vi "Athena Command Main v3.vi"() -> ()   [LabVIEW 2009]
uses:
  UDP3-GPS, INS/UDP 3.ctl
  UDP3-GPS, INS/UDP3rtglob.vi
  <vilib>/userDefined/High Color/nirio_resource_hc.ctl
  <vilib>/rvi/interface/nirviOpenFPGA/nirviOpenFPGA.xnode
  FPGA Bitfiles/Athena Brain.lvproj_FPGA Target 2_FPGA Main.vi.lvbitx
  <vilib>/FPGAPlugInAG/sbRIO-9642/nirviIntfOpen_sbRIO-9642.vi
  <vilib>/rvi/interface/nirviReadWriteControl/nirviReadWriteControl.xnode
  <vilib>/Utility/error.llb/Error Cluster From Error Code.vi
  <vilib>/rvi/errors/niLvFpgaAdjustHostInterfaceError.vi
  <vilib>/rvi/interface/common/niFpgaNodeNameForErrorReporting.ctl
  <vilib>/rvi/errors/niLvFpgaWhatHappensToTopLevelVI.ctl
  <vilib>/LabVIEW Targets/FPGA/RIO/nirio_HostInterface/nirio_ReadBig.vi
  <vilib>/rvi/interface/nirviCloseFPGA/nirviCloseFPGA.xnode
  <vilib>/FPGAPlugInAG/sbRIO-9642/nirviIntfClose_sbRIO-9642.vi
  NiRioSrv.dll
panel:
  out "UDP 3":T1
  in  "Waypoints":cluster{"Latitude":dbl, "Longitude":dbl}[](array[cluster])=[{"Latitude"=42.294143531505355, "Longitude"=-71.26439183950424}, {"Latitude"=42.294083018570596, "Longitude"=-71.2644910812378}, {"Latitude"=42.2940443299425, "Longitude"=-71.2644575536251}, {"Latitude"=42.29408698663367, "Longitude"=-71.26439049839973}]
  out "Heartbeat":bool
  in  "Waypoint Heading":i8
  in  "stop":bool
  in  "Autonomus?":bool=TRUE
  in  "Steering Position Offset":i32
  in  "Steering Control Gain":fxp<+/-,20,5>=0.149993896484375 format="%.17g"
  out "Steering Enabled":bool
  out "Drive Enabled":bool
  out "Speed":dbl(knob) scale=0.0..10.0
  out "Meter":i32(knob) scale=-35.0..35.0
  in  "Tab Control":enum32{"Human Control", "Autonomous"}(tab)=enum."Autonomous"
  in  "Drive Enable":bool
  in  "Steering Enable":bool
  in  "Drive Speed Current (1-3.5)":fxp<+/-,18,8> format="%.13g"
  in  "Steering Position Target":i32
  out "Drive Encoder ft/sec":fxp<+/-,18,8> format="%.13g"
  out "Drivable Paths":T2(graph)
  out "obstacle driveable path lengths":u16[](array[numeric])
  out "line driveable path lengths":u16[](array[numeric])
  in  "min obstacle dist":u16
  in  "paths to graph":enum16{"lines", "obstacles", "both"}(ring)
  in  "Auton Drive Speed Current":fxp<+/-,18,8> format="%.13g"
  in  "obstacle proximity":i16=400
  in  "line proximity":i16=100
  out "Current Heading":cluster{"Lat":dbl, "Longe":dbl, "heading":dbl}
  in  "Override Objective Direction":i8=35
  in  "Use Both Vision and Obstacles":bool
  in  "Display Graph":bool=TRUE
  # "Autonomous"
  # "Human Control"
  # "-35"
  # "-30"
  # "-25"
  # "-20"
  # "-15"
  # "-10"
  # "-5"
  # "-1"
  # "1"
  # "5"
  # "10"
  # "15"
  # "20"
  # "25"
  # "30"
  # "35"
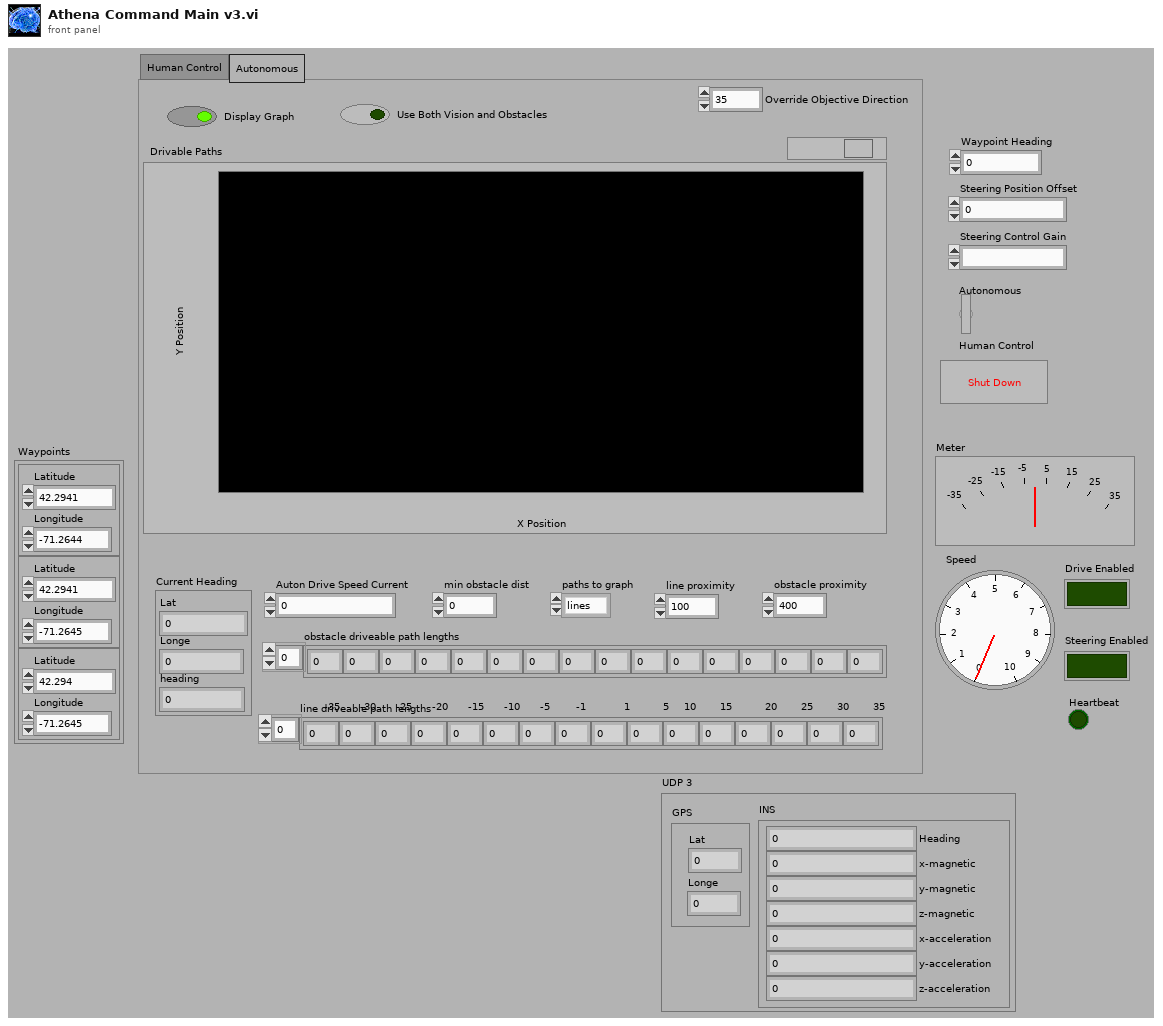
[diagram p1: front panel]
types:
  T1 = typedef "UDP 3.ctl" = cluster{"GPS":cluster{"Lat":dbl, "Longe":dbl}, "INS":cluster{"Heading":dbl, "x-magnetic":dbl, "y-magnetic":dbl, "z-magnetic":dbl, "x-acceleration":dbl, "y-acceleration":dbl, "z-acceleration":dbl}}
  T2 = cluster{"New X Position":i16, "New Y Position":i16}[]
  T3 = typedef "nirio_resource_hc.ctl" = tag
  T4 = typedef "niFpgaNodeNameForErrorReporting.ctl" = enum16{"Open FPGA VI Reference", "Read/Write Control", "Invoke Method: Abort", "Invoke Method: Acknowledge IRQ", "Invoke Method: Download", "Invoke Method: FIFO.Configure", "Invoke Method: FIFO.Read", "Invoke Method: FIFO.Start", "Invoke Method: FIFO.Stop", "Invoke Method: FIFO.Write", "Invoke Method: Reset", "Invoke Method: Run", "Invoke Method: Wait on IRQ", "Close FPGA VI Reference"}
  T5 = typedef "niLvFpgaWhatHappensToTopLevelVI.ctl" = enum16{"top level VI scripted behind XNode", "top level VI inlined behind XNode"}
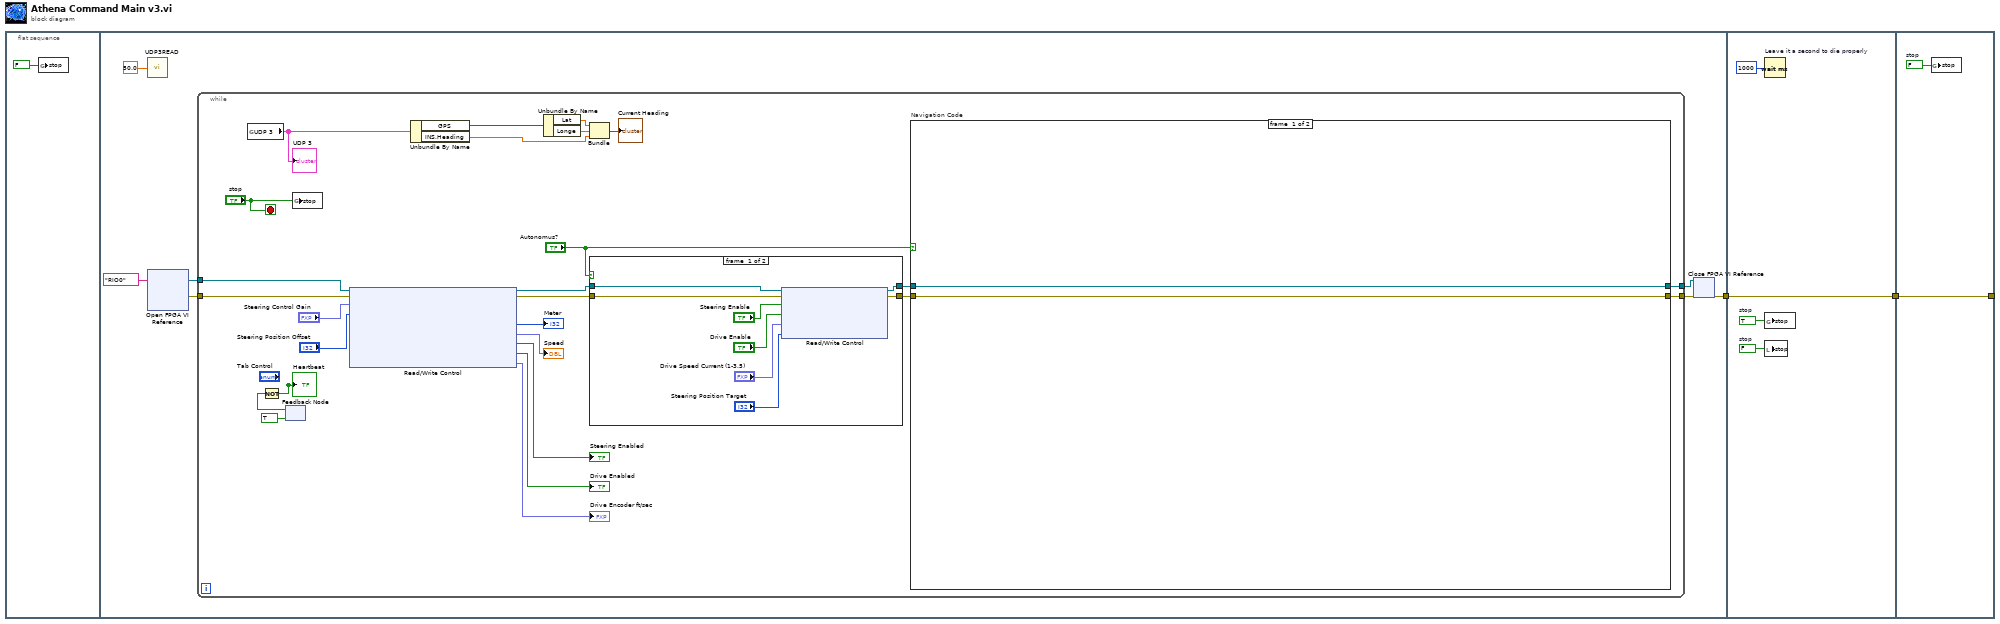
[diagram p0: block diagram]
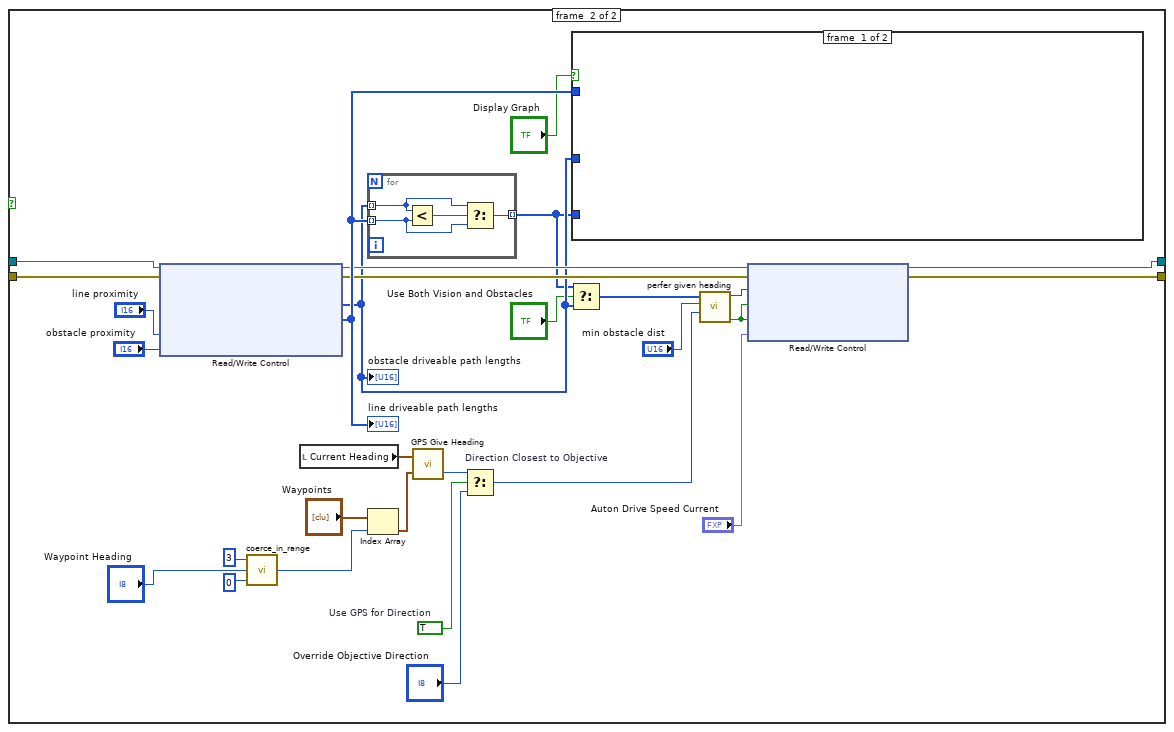
[diagram p2: hidden frame]
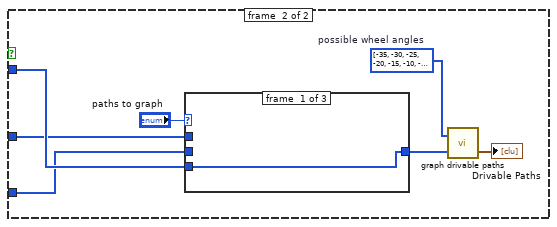
[diagram p3: hidden frame]
diagram:
  n1 = flat-sequence {
    tunnel: [w5] -> w2
    tunnel: w2 -> [w620]
    tunnel: [w620] -> w1
    tunnel: [w625] -> _
    tunnel: w1 -> [w625]
    frame #0 {
      n2 = global write "UDP3rtglob.vi" "stop"(FALSE ("stop")) -> ()
    }
    frame #1 {
      n3 = call "UDP3READ.vi"("Frequency, in Hz"=50.0) -> ()
      n4 = xnode "Open FPGA VI Reference"("resource name"=T3 "RIO0") -> ("FPGA VI Reference Out"=w10:refnum<k20>, "error out"=w7:errorcluster)  [unwired: 1 in]
      n5 = while {
        tunnel: w10 -> [w44]
        tunnel: w7 -> [w25]
        tunnel: [w34] -> w9
        tunnel: [w33] -> w6
        stop <- "stop" stop-if-true
        n6 = global read "UDP3rtglob.vi" "UDP 3"() -> (w19:T1)
        "UDP 3" <- w19
        n7 = feedback #1(TRUE) -> (w27:bool)
        n8 = Not(x=w27) -> (.not. x?=w26:bool)
        "Heartbeat" <- w26
        n9 = global write "UDP3rtglob.vi" "stop"("stop") -> ()
        n10 = xnode "Read/Write Control"("FPGA VI Reference In"=w44, "error in"=w25, "Steering Proportional Control Feedback Gain"="Steering Control Gain", "Steering Position Offset"="Steering Position Offset") -> ("FPGA VI Reference Out"=w43:refnum<k20>, "error out"=w42:errorcluster, "Steering Position"=→"Meter":i32, "Drive Speed Current"=→"Speed":fxp<+/-,18,8>, "Steering Enabled?"=→"Steering Enabled":bool, "Drive Enabled?"=→"Drive Enabled":bool, "Drive Encoder ft/sec"=→"Drive Encoder ft/sec":fxp<+/-,18,8>)
        n11 = Unbundle By Name(w19) -> ("GPS"=w20:cluster{"Lat":dbl, "Longe":dbl}, "INS.Heading"=w24:dbl)
        n12 = Unbundle By Name(w20) -> ("Lat"=w21:dbl, "Longe"=w22:dbl)
        n13 = Bundle("Lat"=w21, "Longe"=w22, "Heading"=w24) -> (→"Current Heading":cluster{"Lat":dbl, "Longe":dbl, "Heading":dbl})  [unwired: 1 in]
        n14 = case shown="False" "Autonomus?" {
          tunnel: w43 -> [w312 w417]
          tunnel: w42 -> [w305 w416]
          tunnel: [w307 w416] -> w41
          tunnel: [w306 w417] -> w40
          frame #0 {
            n15 = xnode "Read/Write Control"("FPGA VI Reference In"=w312, "error in"=w305, "Enable Steering"="Steering Enable", "Enable Drive"="Drive Enable", "Drive Speed Current (1-3.5)"="Drive Speed Current (1-3.5)", "Steering Position Target"="Steering Position Target") -> ("FPGA VI Reference Out"=w306:refnum<k20>, "error out"=w307:errorcluster)
          }
          frame #1 {
          }
        }
        n16 = case "Navigation Code" shown="True" "Autonomus?" {
          tunnel: w41 -> [w45 w51]
          tunnel: w40 -> [w46 w75]
          tunnel: [w46 w68] -> w34
          tunnel: [w45 w69] -> w33
          frame #0 {
          }
          frame #1 {
            w48 = TRUE  # Use GPS for Direction
            n17 = xnode "Read/Write Control"("FPGA VI Reference In"=w75, "error in"=w51, "line proximity"="line proximity", "obstacle proximity"="obstacle proximity") -> ("FPGA VI Reference Out"=w72:refnum<k20>, "error out"=w71:errorcluster, "obstacle driveable path lengths"=w58:u16[], "line driveable path lengths"=w73:u16[])  [unwired: 1 in]
            "obstacle driveable path lengths" <- w58
            "line driveable path lengths" <- w73
            n18 = call "coerce_in_range.vi"("min"=i8 0, "x"="Waypoint Heading", "max"=i8 3) -> ("coerced x"=w59:i8)  [unwired: 2 in]
            n19 = local read "Current Heading"() -> (w47:cluster{"Lat":dbl, "Longe":dbl, "heading":dbl})
            n20 = for {
              tunnel: w58 -> [w191] mode=indexing
              tunnel: w73 -> [w190] mode=indexing
              tunnel: [w189] -> w52 mode=indexing
              n21 = Less?(x=w191, y=w190) -> (x < y?=w192:bool)
              n22 = Select(t=w191, s=w192, f=w190) -> (s? t:f=w189:u16)
            }
            n23 = Index Array(array="Waypoints", index=w59) -> (element=w63:cluster{"Latitude":dbl, "Longitude":dbl})
            n24 = call "GPS Give Heading.vi"("Target Position"=w63, "Current State"=w47) -> ("Wheel Angle"=w56:i8)  [unwired: 1 out]
            n25 = Select "Direction Closest to Objective"(t=w56, s=w48, f="Override Objective Direction") -> (s? t:f=w50:i8)
            n26 = Select(t=w52, s="Use Both Vision and Obstacles", f=w58) -> (s? t:f=w55:u16[])
            n27 = case shown="False" "Display Graph" {
              tunnel: w73 -> [_ w82]
              tunnel: w58 -> [_ w81]
              tunnel: w52 -> [_ w76]
              frame #0 {
              }
              frame #1 {
                w80 = i8[] [-35, -30, -25, -20, -15, -10, -5, -1, 1, 5, 10, 15, 20, 25, 30, 35]  # possible wheel angles
                n28 = case shown="\"both\"" "paths to graph" {
                  tunnel: w76 -> [_ _ w85]
                  tunnel: w81 -> [_ w84 _]
                  tunnel: w82 -> [w83 _ _]
                  tunnel: [w83 w84 w85] -> w77
                  frame #0 {
                  }
                  frame #1 {
                  }
                  frame #2 {
                  }
                }
                n29 = call "graph drivable paths.vi"("updated max path lengths"=w77, "possible wheel angles"=w80) -> ("XY Graph"=→"Drivable Paths":T2)  [unwired: 1 in]
              }
            }
            n30 = call "perfer given heading.vi"("desired heading"=w50, "min obstacle dist"="min obstacle dist", "driveable path lengths"=w55) -> ("driveable paths?"=w57:bool, "wheel angle"=w70:i8)  [unwired: 7 in]
            n31 = xnode "Read/Write Control"("FPGA VI Reference In"=w72, "error in"=w71, "Steering Position Target"=w70, "Enable Drive"=w57, "Enable Steering"=w57, "Drive Speed Current (1-3.5)"="Auton Drive Speed Current") -> ("FPGA VI Reference Out"=w68:refnum<k20>, "error out"=w69:errorcluster)
          }
        }
      }
      n32 = xnode "Close FPGA VI Reference"("FPGA VI Reference In"=w9, "error in"=w6) -> ("error out"=w5:errorcluster)
    }
    frame #2 {
      w622 = TRUE  # stop
      w623 = FALSE  # stop
      n33 = Wait (ms) "Leave it a second to die properly"(milliseconds to wait=u32 1000) -> ()  [unwired: 1 out]
      n34 = global write "UDP3rtglob.vi" "stop"(w622) -> ()
      n35 = local write "stop"(w623) -> ()
    }
    frame #3 {
      w624 = FALSE  # stop
      n36 = global write "UDP3rtglob.vi" "stop"(w624) -> ()
    }
  }
